vi "DBO_Init.vi"(1 "base path":path=path "D:/yan/yan2015A/Hysteresis1/DiscreteBacklashModel/DBO_Para") -> (0 "DBO_Para":T1)   [LabVIEW 2011]
uses:
  <vilib>/Utility/file.llb/Read From Spreadsheet File (DBL).vi
panel:
  out "K":dbl
  out "y0":dbl
  out "x0":dbl
  out "size(s) 2":i32[](array[numeric])
  out "H size(s) 4":i32[](array[numeric])
  out "S Inv":dbl[][](array[numeric])
  out "H size(s) 3":i32[](array[numeric])
  out "H Inv":dbl[][](array[numeric])
  out "size(s)":i32[](array[numeric])
  out "H size(s) 2":i32[](array[numeric])
  out "S":dbl[][](array[numeric])
  out "H size(s)":i32[](array[numeric])
  out "H":dbl[][](array[numeric])
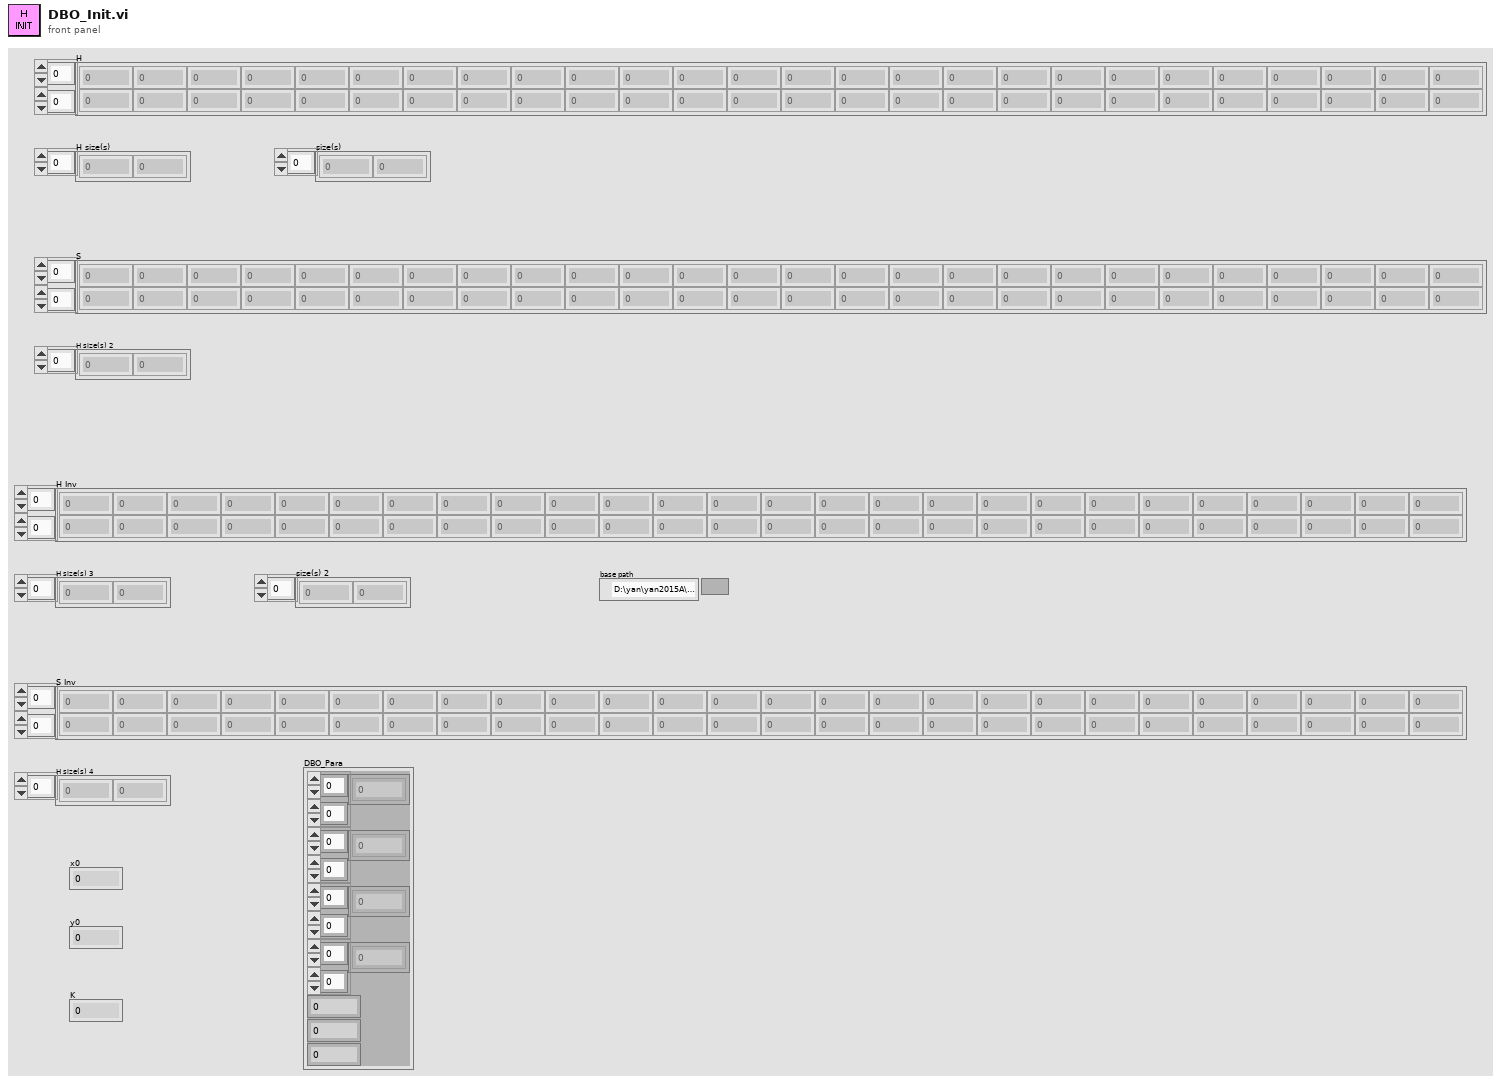
[diagram p1: front panel]
types:
  T1 = cluster{dbl[][], dbl[][], dbl[][], dbl[][], dbl, dbl, dbl}
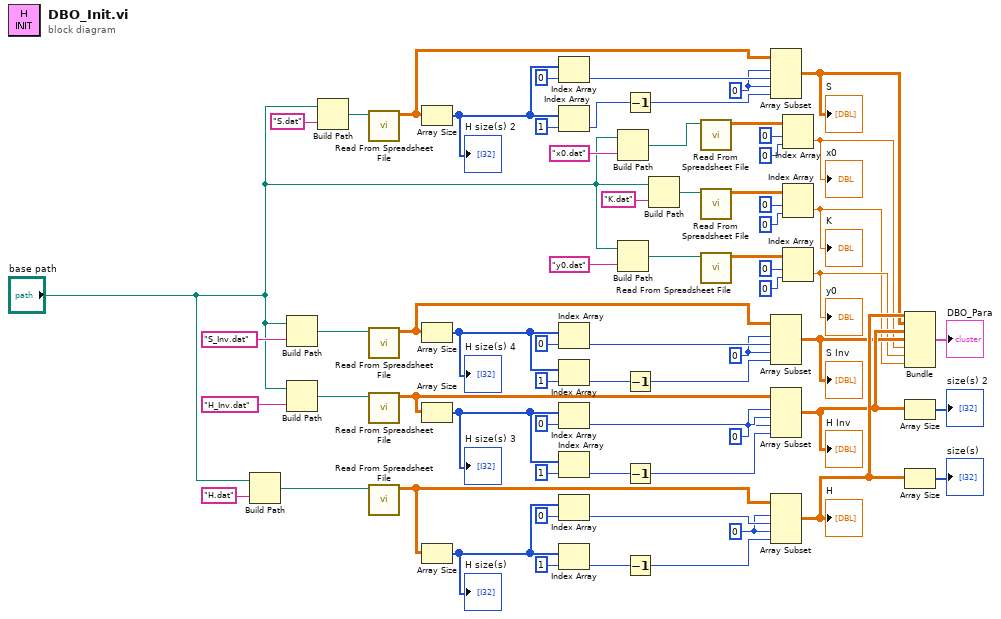
[diagram p0: block diagram]
diagram:
  w30 = 0 ("index")
  w40 = 0 ("index")
  w51 = 0 ("index")
  w61 = 0 ("index")
  n1 = Build Path(base path="base path", name or relative path="H.dat") -> (appended path=w65:path)
  n2 = Build Path(base path="base path", name or relative path="S_Inv.dat") -> (appended path=w34:path)
  n3 = Build Path(base path="base path", name or relative path="H_Inv.dat") -> (appended path=w44:path)
  n4 = Build Path(base path="base path", name or relative path="S.dat") -> (appended path=w55:path)
  n5 = call-poly <vilib>:"Read From Spreadsheet File.vi"("file path (dialog if empty)"=w55) -> ("all rows"=w54:dbl[][])  [unwired: 6 in, 4 out]
  n6 = call-poly <vilib>:"Read From Spreadsheet File.vi"("file path (dialog if empty)"=w34) -> ("all rows"=w33:dbl[][])  [unwired: 6 in, 4 out]
  n7 = call-poly <vilib>:"Read From Spreadsheet File.vi"("file path (dialog if empty)"=w44) -> ("all rows"=w43:dbl[][])  [unwired: 6 in, 4 out]
  n8 = call-poly <vilib>:"Read From Spreadsheet File.vi"("file path (dialog if empty)"=w65) -> ("all rows"=w64:dbl[][])  [unwired: 6 in, 4 out]
  n9 = Array Size(array=w54) -> (size(s)=w50:i32[])
  "H size(s) 2" <- w50
  n10 = Array Size(array=w33) -> (size(s)=w29:i32[])
  "H size(s) 4" <- w29
  n11 = Array Size(array=w43) -> (size(s)=w39:i32[])
  "H size(s) 3" <- w39
  n12 = Array Size(array=w64) -> (size(s)=w60:i32[])
  "H size(s)" <- w60
  n13 = Index Array(array=w50, index=0) -> (element=w52:i32)
  n14 = Index Array(array=w50, index=1) -> (element=w48:i32)
  n15 = Index Array(array=w29, index=0) -> (element=w31:i32)
  n16 = Index Array(array=w29, index=1) -> (element=w27:i32)
  n17 = Index Array(array=w39, index=0) -> (element=w41:i32)
  n18 = Index Array(array=w39, index=1) -> (element=w37:i32)
  n19 = Index Array(array=w60, index=0) -> (element=w62:i32)
  n20 = Index Array(array=w60, index=1) -> (element=w58:i32)
  n21 = Build Path(base path="base path", name or relative path="x0.dat") -> (appended path=w23:path)
  n22 = Build Path(base path="base path", name or relative path="y0.dat") -> (appended path=w18:path)
  n23 = Decrement(x=w48) -> (x-1=w47:i32)
  n24 = Decrement(x=w27) -> (x-1=w26:i32)
  n25 = Decrement(x=w37) -> (x-1=w36:i32)
  n26 = Decrement(x=w58) -> (x-1=w57:i32)
  n27 = Build Path(base path="base path", name or relative path="K.dat") -> (appended path=w13:path)
  n28 = call-poly <vilib>:"Read From Spreadsheet File.vi"("file path (dialog if empty)"=w23) -> ("all rows"=w22:dbl[][])  [unwired: 6 in, 4 out]
  n29 = call-poly <vilib>:"Read From Spreadsheet File.vi"("file path (dialog if empty)"=w13) -> ("all rows"=w12:dbl[][])  [unwired: 6 in, 4 out]
  n30 = call-poly <vilib>:"Read From Spreadsheet File.vi"("file path (dialog if empty)"=w18) -> ("all rows"=w17:dbl[][])  [unwired: 6 in, 4 out]
  n31 = Array Subset(array=w54, index (row)=w51, length (row)=w52, index (col)=w51, length (col)=w47) -> (w8:dbl[][])
  "S" <- w8
  n32 = Array Subset(array=w33, index (row)=w30, length (row)=w31, index (col)=w30, length (col)=w26) -> (w6:dbl[][])
  "S Inv" <- w6
  n33 = Array Subset(array=w43, index (row)=w40, length (row)=w41, index (col)=w40, length (col)=w36) -> (w7:dbl[][])
  "H Inv" <- w7
  n34 = Array Subset(array=w64, index (row)=w61, length (row)=w62, index (col)=w61, length (col)=w57) -> (w9:dbl[][])
  "H" <- w9
  n35 = Index Array(array=w22, index (row)=0, index (col)=0 ("disabled index (col)")) -> (element=w5:dbl)
  "x0" <- w5
  n36 = Index Array(array=w12, index (row)=0, index (col)=0 ("disabled index (col)")) -> (element=w3:dbl)
  "K" <- w3
  n37 = Index Array(array=w17, index (row)=0, index (col)=0 ("disabled index (col)")) -> (element=w4:dbl)
  "y0" <- w4
  n38 = Bundle(w9, w8, w7, w6, w5, w4, w3) -> (→"DBO_Para":T1)  [unwired: 1 in]
  n39 = Array Size(array=w7) -> (size(s)=→"size(s) 2":i32[])
  n40 = Array Size(array=w9) -> (size(s)=→"size(s)":i32[])
